vi "repump_cleaning.vi"(4 "BG indexes":i32[](array[numeric]), 5 "first elyse clock count":dbl, 6 "repump_values IN":T1, 7 "repump_correction":bool, 8 "repump_limits":T3, 9 "II channel in":cluster{"BG":sgl[], "Ie":sgl[], "I0":sgl[]}[](array[cluster]), 10 "I channel in":cluster{"BG":sgl[], "Ie":sgl[], "I0":sgl[]}[](array[cluster])) -> (2 "II channel out":cluster{"BG":sgl[], "Ie":sgl[], "I0":sgl[]}[](array[cluster]), 3 "I channel out":cluster{"BG":sgl[], "Ie":sgl[], "I0":sgl[]}[](array[cluster]))   [LabVIEW 2020, in "Detector.lvclass"]
uses:
  Detector.lvclass
  dependecies/ControlsVIs/Clusters-def/Def_repump_limits.ctl
  def_repump_values_array.ctl
  Oscilloscope/def_repump_value.ctl
  Oscilloscope/Oscilloscope.lvclass
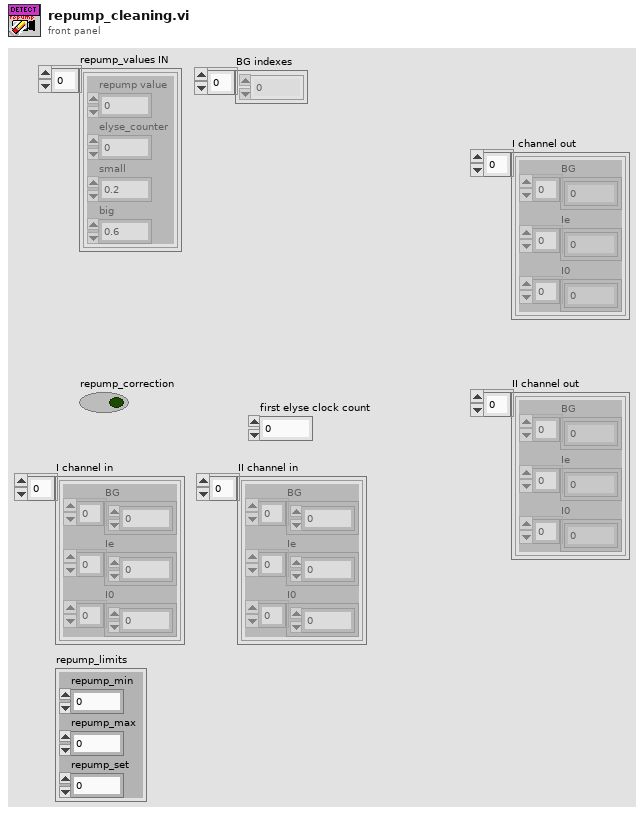
[diagram p1: front panel]
types:
  T1 = typedef "def_repump_values_array.ctl" = T2[]
  T2 = typedef "def_repump_value.ctl" = cluster{"repump value":dbl, "elyse_counter":i64, "small":dbl, "big ":dbl}
  T3 = typedef "Oscilloscope.lvclass/Def_repump_limits.ctl" = cluster{"repump_min":dbl, "repump_max":dbl, "repump_set":dbl}
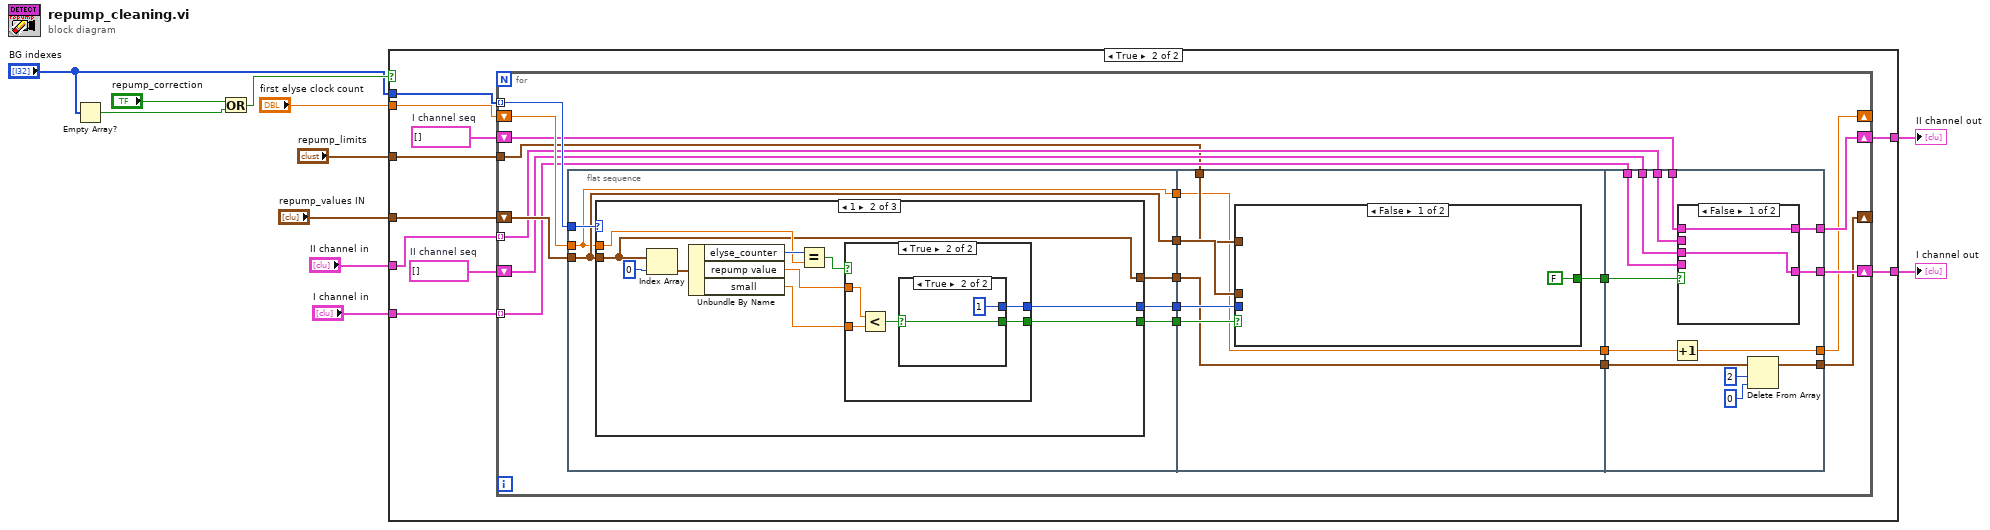
[diagram p0: block diagram]
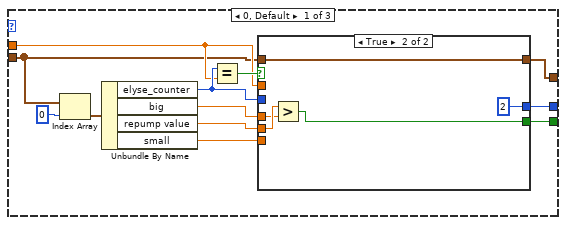
[diagram p3: hidden frame]
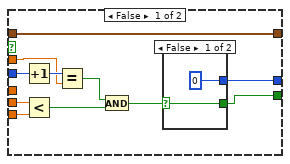
[diagram p4: hidden frame]
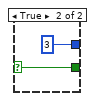
[diagram p5: hidden frame]
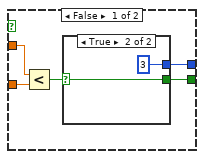
[diagram p6: hidden frame]
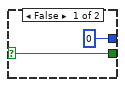
[diagram p7: hidden frame]
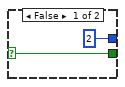
[diagram p8: hidden frame]
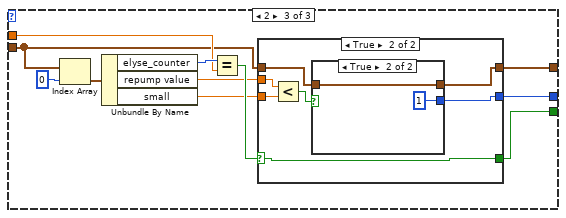
[diagram p9: hidden frame]
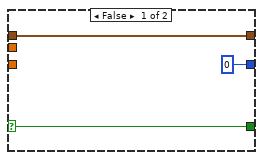
[diagram p10: hidden frame]
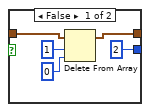
[diagram p11: hidden frame]
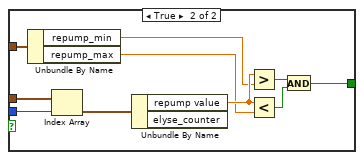
[diagram p12: hidden frame]
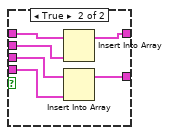
[diagram p13: hidden frame]
diagram:
  n1 = Empty Array?(array="BG indexes") -> (empty?=w5:bool)
  n2 = Or(x="repump_correction", y=w5) -> (x .or. y?=w3:bool)
  n3 = case shown="True" w3 {
    tunnel: [w13 w18] -> w6
    tunnel: "I channel in" -> [w13 w20]
    tunnel: [w12 w19] -> w7
    tunnel: "II channel in" -> [w12 w21]
    tunnel: "repump_values IN" -> [_ w17]
    tunnel: "repump_limits" -> [_ w15]
    tunnel: "BG indexes" -> [_ w14]
    tunnel: "first elyse clock count" -> [_ w16]
    frame False {
    }
    frame True {
      w22 = cluster{"BG":i32[], "Ie":i32[], "I0":i32[]}[] []  # II channel seq
      w23 = cluster{"BG":i32[], "Ie":i32[], "I0":i32[]}[] []  # I channel seq
      n4 = for {
        shift-right: [w34] -> w18
        shift-left: w22 -> [w38]
        shift-right: [w35] -> w19
        shift-left: w23 -> [w39]
        tunnel: w21 -> [w36] mode=indexing
        tunnel: w20 -> [w37] mode=indexing
        tunnel: w14 -> [w42] mode=indexing
        tunnel: w15 -> [w32]
        shift-right: [w29] -> _
        shift-left: w16 -> [w41]
        shift-right: [w24] -> _
        shift-left: w17 -> [w43]
        n5 = flat-sequence {
          tunnel: w43 -> [w48]
          tunnel: w42 -> [w49]
          tunnel: w41 -> [w45]
          tunnel: [w48] -> w33
          tunnel: [w47] -> w31
          tunnel: [w46] -> w30
          tunnel: [w45] -> w27
          tunnel: [w44] -> w25
          tunnel: [w143] -> w40
          tunnel: w33 -> [w144]
          tunnel: w32 -> [w142]
          tunnel: w31 -> [w141]
          tunnel: w30 -> [w140]
          tunnel: [w139] -> w28
          tunnel: w27 -> [w139]
          tunnel: [w138] -> w26
          tunnel: w25 -> [w138]
          tunnel: w40 -> [w168]
          tunnel: w39 -> [w167]
          tunnel: w38 -> [w166]
          tunnel: w37 -> [w165]
          tunnel: w36 -> [w164]
          tunnel: [w163] -> w35
          tunnel: [w162] -> w34
          tunnel: [w160] -> w29
          tunnel: w28 -> [w161]
          tunnel: w26 -> [w159]
          tunnel: [w158] -> w24
          frame #0 {
            n6 = case shown="1" w49 {
              tunnel: w48 -> [w51 w82 w111]
              tunnel: w45 -> [w53 w88 w117]
              tunnel: [w56 w86 w115] -> w47
              tunnel: [w55 w83 w112] -> w46
              tunnel: [w50 w82 w110] -> w44
              frame 0, Default {
                n7 = Index Array(array=w51, index=0) -> (element=w60:T2)
                n8 = Unbundle By Name(w60) -> ("elyse_counter"=w54:i64, "big"=w57:dbl, "repump value"=w58:dbl, "small"=w52:dbl)
                n9 = Equal?(x=w54, y=w53) -> (x = y?=w59:bool)
                n10 = case shown="True" w59 {
                  tunnel: w58 -> [w69 w81]
                  tunnel: w57 -> [_ w80]
                  tunnel: [w63 w79] -> w56
                  tunnel: [w64 2] -> w55
                  tunnel: w54 -> [w72 _]
                  tunnel: w53 -> [w70 _]
                  tunnel: w52 -> [w68 _]
                  tunnel: w51 -> [w62 w77]
                  tunnel: [w62 w77] -> w50
                  frame False {
                    n11 = Increment(x=w72) -> (x+1=w71:i64)
                    n12 = Less?(x=w69, y=w68) -> (x < y?=w66:bool)
                    n13 = Equal?(x=w71, y=w70) -> (x = y?=w67:bool)
                    n14 = And(x=w67, y=w66) -> (x .and. y?=w65:bool)
                    n15 = case shown="False" w65 {
                      selector: w65 -> [w74 w75]
                      tunnel: [0 3] -> w64
                      tunnel: [w74 w75] -> w63
                      frame False {
                      }
                      frame True {
                      }
                    }
                  }
                  frame True {
                    n16 = Greater?(x=w81, y=w80) -> (0:w79:bool)
                  }
                }
              }
              frame 1 {
                n17 = Index Array(array=w82, index=0) -> (element=w90:T2)
                n18 = Unbundle By Name(w90) -> ("elyse_counter"=w89:i64, "repump value"=w85:dbl, "small"=w84:dbl)
                n19 = Equal?(x=w89, y=w88) -> (x = y?=w87:bool)
                n20 = case shown="True" w87 {
                  tunnel: [w92 w101] -> w86
                  tunnel: w85 -> [w96 w105]
                  tunnel: w84 -> [w95 w104]
                  tunnel: [w93 w102] -> w83
                  frame False {
                    n21 = Less?(x=w96, y=w95) -> (x < y?=w94:bool)
                    n22 = case shown="True" w94 {
                      selector: w94 -> [w97 w99]
                      tunnel: [0 3] -> w93
                      tunnel: [w97 w99] -> w92
                      frame False {
                      }
                      frame True {
                      }
                    }
                  }
                  frame True {
                    n23 = Less?(x=w105, y=w104) -> (x < y?=w103:bool)
                    n24 = case shown="True" w103 {
                      selector: w103 -> [w106 w108]
                      tunnel: [2 1] -> w102
                      tunnel: [w106 w108] -> w101
                      frame False {
                      }
                      frame True {
                      }
                    }
                  }
                }
              }
              frame 2 {
                n25 = Index Array(array=w111, index=0) -> (element=w119:T2)
                n26 = Unbundle By Name(w119) -> ("elyse_counter"=w118:i64, "repump value"=w114:dbl, "small"=w113:dbl)
                n27 = Equal?(x=w118, y=w117) -> (x = y?=w116:bool)
                n28 = case shown="True" w116 {
                  selector: w116 -> [w123 w127]
                  tunnel: [w123 w127] -> w115
                  tunnel: w114 -> [_ w130]
                  tunnel: w113 -> [_ w129]
                  tunnel: [0 w126] -> w112
                  tunnel: w111 -> [w121 w125]
                  tunnel: [w121 w124] -> w110
                  frame False {
                  }
                  frame True {
                    n29 = Less?(x=w130, y=w129) -> (x < y?=w128:bool)
                    n30 = case shown="True" w128 {
                      tunnel: [2 1] -> w126
                      tunnel: w125 -> [w134 w136]
                      tunnel: [w133 w136] -> w124
                      frame False {
                        n31 = Delete From Array(array=w134, length=1, index=0) -> (array with subset deleted=w133:T1)  [unwired: 1 out]
                      }
                      frame True {
                      }
                    }
                  }
                }
              }
            }
          }
          frame #1 {
            n32 = case shown="False" w141 {
              tunnel: w144 -> [_ w151]
              tunnel: [FALSE w150] -> w143
              tunnel: w142 -> [_ w149]
              tunnel: w140 -> [_ w146]
              frame False {
              }
              frame True {
                n33 = Unbundle By Name(w149) -> ("repump_min"=w148:dbl, "repump_max"=w147:dbl)
                n34 = Index Array(array=w151, index=w146) -> (element=w155:T2)
                n35 = Unbundle By Name(w155) -> ("repump value"=w154:dbl)  [unwired: 1 out]
                n36 = Greater?(x=w154, y=w148) -> (0:w152:bool)
                n37 = Less?(x=w154, y=w147) -> (x < y?=w153:bool)
                n38 = And(x=w152, y=w153) -> (x .and. y?=w150:bool)
              }
            }
          }
          frame #2 {
            n39 = Increment(x=w161) -> (x+1=w160:dbl)
            n40 = case shown="False" w168 {
              tunnel: w167 -> [w170 w176]
              tunnel: [w170 w175] -> w163
              tunnel: [w169 w173] -> w162
              tunnel: w166 -> [w169 w174]
              tunnel: w165 -> [_ w172]
              tunnel: w164 -> [_ w171]
              frame False {
              }
              frame True {
                n41 = Insert Into Array(array=w176, new element=w171) -> (w175:cluster{"BG":i32[], "Ie":i32[], "I0":i32[]}[])  [unwired: 1 in]
                n42 = Insert Into Array(array=w174, new element=w172) -> (w173:cluster{"BG":i32[], "Ie":i32[], "I0":i32[]}[])  [unwired: 1 in]
              }
            }
            n43 = Delete From Array(array=w159, length=2, index=0) -> (array with subset deleted=w158:T1)  [unwired: 1 out]
          }
        }
      }
    }
  }
  "II channel out" <- w7
  "I channel out" <- w6
